vi "Settings.vi"(6 "Particle Measurements (Pixels) (Particle Analysis 1) 3":dbl[](array[numeric]), 7 "Numeric":i32, 9 "Particle Measurements (Pixels) (Particle Analysis 1) 2":dbl[](array[numeric]), 10 "Particle Measurements (Pixels) (Particle Analysis 1)":dbl[](array[numeric]), 11 "Refnum in":T2) -> (1 "Iter":i32, 2 "Cluster":T1, 3 "Refnum out":T2)   [LabVIEW 2020]
uses:
  <vilib>/vision/Image Controls.llb/IMAQ Image.ctl
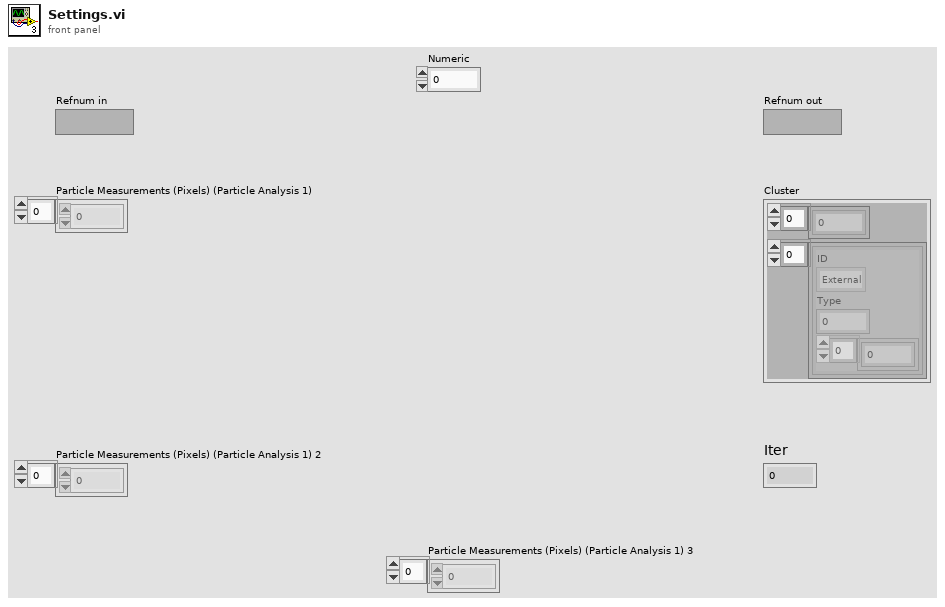
[diagram p1: front panel]
types:
  T1 = cluster{i32[], cluster{"ID":enum32{"External", "Internal"}, "Type":u32, i32[]}[]}
  T2 = typedef "IMAQ Image.ctl" = refnum<image>
  T3 = cluster{"ID":enum32{"External", "Internal"}, "Type":u32, i32[]}
  T4 = cluster{"ID":enum32{"External", "Internal"}, "Type":u32, i32[]}[]
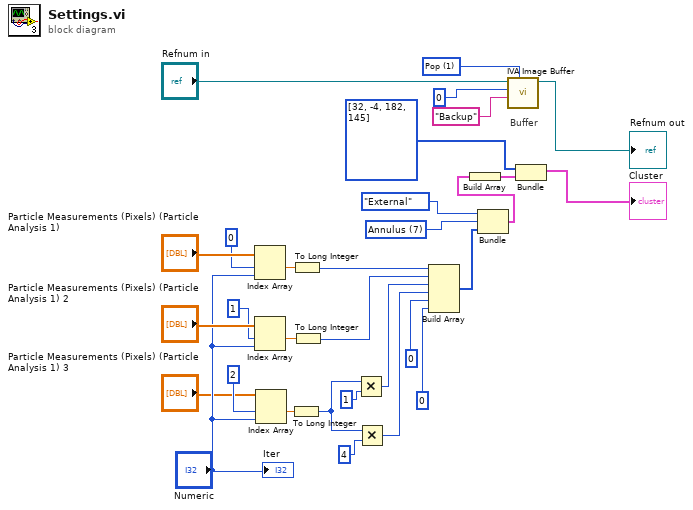
[diagram p0: block diagram]
diagram:
  w27 = u16 1 items=["Push", "Pop", "Reset"] ("Function")
  w12 = u32 7 items=["No Selection", "Point", "Line", "Rectangle", "Oval", "Polygon", "Freehand Region", "Annulus", "Unused2", "Unused3", "Broken Line", "Freehand Line", "Rotated Rectangle"] ("Type")
  # "Buffer"
  n1 = Index Array(array="Particle Measurements (Pixels) (Particle Analysis 1)", index #1=0 ("disabled index (col)"), index #2="Numeric") -> (element #1=w3:dbl)  [unwired: 1 out]
  n2 = Index Array(array="Particle Measurements (Pixels) (Particle Analysis 1) 2", index #1=1 ("disabled index (col)"), index #2="Numeric") -> (element #1=w2:dbl)  [unwired: 1 out]
  n3 = Index Array(array="Particle Measurements (Pixels) (Particle Analysis 1) 3", index #1=2 ("disabled index (col)"), index #2="Numeric") -> (element #1=w1:dbl)  [unwired: 1 out]
  n4 = To Long Integer(number=w1) -> (32bit integer=w6:i32)
  n5 = To Long Integer(number=w3) -> (32bit integer=w4:i32)
  n6 = To Long Integer(number=w2) -> (32bit integer=w5:i32)
  n7 = Multiply(x=w6, y=1) -> (x*y=w9:i32)
  n8 = Multiply(x=w6, y=4) -> (x*y=w10:i32)
  n9 = Build Array(w4, w5, w9, w10, 0 ("element"), 0 ("element")) -> (w13:i32[])
  n10 = Bundle("ID"=enum32{"External", "Internal"}."External", "Type"=w12, w13) -> (w14:T3)  [unwired: 1 in]
  n11 = Build Array(w14) -> (w18:T4)
  n12 = call <vilib>:"IVA Image Buffer.vi"("Function"=w27, "Prefix"="Backup", "Buffer #"=0, "Image In"="Refnum in") -> ("Image Out"=→"Refnum out":T2)  [unwired: 1 in, 6 out]
  n13 = Bundle(i32[] [32, -4, 182, 145], w18) -> (→"Cluster":T1)  [unwired: 1 in]
  "Iter" <- "Numeric"
